vi "Test_meas_mode_status.vi"() -> ()   [LabVIEW 2019]
uses:
  D:/SOFT_REPO_GUM/renishawxl80sdk/XL-80_forum DLL/Interop.DX10SDKADAPTORLib.dll
  SOFT_REPO_GUM/renishawxl80sdk/XL-80_forum DLL/Interop.DX10SDKADAPTORLib.dll
panel:
  out "32bit integer":i32
  out "MEASUREMENT_INDETERMINATE":i32(ring) items=["MEASUREMENT_INDETERMINATE", "MEASUREMENT_LINEAR_PLANE", "MEASUREMENT_LINEAR_RETRO", "MEASUREMENT_ANGULAR", "MEASUREMENT_STRAIGHTNESS_SHORT", "MEASUREMENT_STRAIGHTNESS_LONG", "MEASUREMENT_VELOCITY_RETRO"]
  out "x << y":u32
  out "modeMask":u32
  out "status":u32
  out "ML10_MEASUREMENT_MODE":i32(ring)=1 items=["ML10_AVERAGING_ON"=1, "ML10_TPIN_SELECTED"=4, "ML10_BEAM_LOW"=64, "ML10_BEAM_LOSS"=128, "ML10_STABILITY_LOSS"=256, "ML10_PREHEAT"=2048, "ML10_LASER_TOO_COLD"=4096, "ML10_LASER_TOO_HOT"=8192, "ML10_LASER_UNSTABLE"=16384, "ML10_LASER_FAIL"=32768, "ML10_NOT_RESPONDING"=65536, "ML10_LONG_TERM_AVERAGING_ON"=524288, "ML10_MEASUREMENT_MODE"=7340032, "ML10_HIGH_SPEED_ERROR"=8388608, "ML10_DYNAMIC_SELECTED"=16777216]
  out "Status":i32(ring)=1 items=["ML10_AVERAGING_ON"=1, "ML10_TPIN_SELECTED"=4, "ML10_BEAM_LOW"=64, "ML10_BEAM_LOSS"=128, "ML10_STABILITY_LOSS"=256, "ML10_PREHEAT"=2048, "ML10_LASER_TOO_COLD"=4096, "ML10_LASER_TOO_HOT"=8192, "ML10_LASER_UNSTABLE"=16384, "ML10_LASER_FAIL"=32768, "ML10_NOT_RESPONDING"=65536, "ML10_LONG_TERM_AVERAGING_ON"=524288, "ML10_MEASUREMENT_MODE"=7340032, "ML10_HIGH_SPEED_ERROR"=8388608, "ML10_DYNAMIC_SELECTED"=16777216]
  out "pbstrSerNum":string
  out "Connect":bool
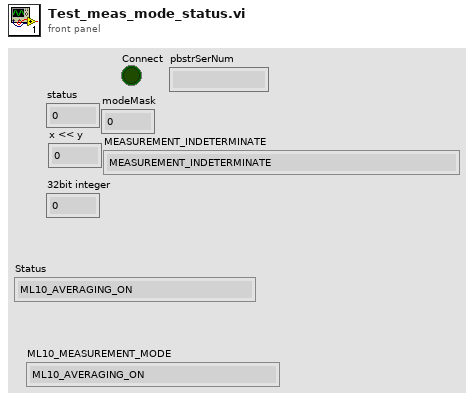
[diagram p1: front panel]
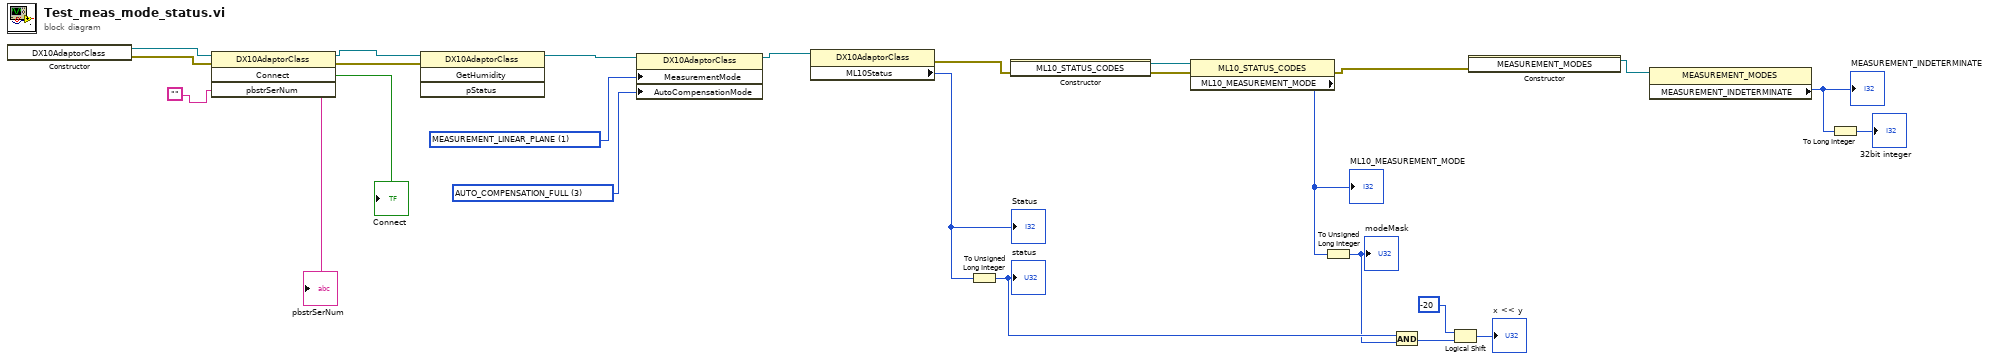
[diagram p0: block diagram]
diagram:
  w18 = 3 items=["AUTO_COMPENSATION_OFF"=0, "AUTO_COMPENSATION_AIR"=1, "AUTO_COMPENSATION_FULL"=3] ("AutoCompensationMode")
  w19 = 1 items=["MEASUREMENT_INDETERMINATE", "MEASUREMENT_LINEAR_PLANE", "MEASUREMENT_LINEAR_RETRO", "MEASUREMENT_ANGULAR", "MEASUREMENT_STRAIGHTNESS_SHORT", "MEASUREMENT_STRAIGHTNESS_LONG", "MEASUREMENT_VELOCITY_RETRO"] ("MeasurementMode")
  n1 = constructor class="DX10AdaptorClass"() -> (reference out=w16:refnum<k24>, error out=w25:errorcluster)  [unwired: 3 in, 1 out]
  n2 = invoke class="DX10AdaptorClass" method="Connect"(reference=w16, error in=w25, "pbstrSerNum"="") -> (reference out=w15:refnum<k24>, error out=w21:errorcluster, "Connect"=→"Connect":bool, "pbstrSerNum"=→"pbstrSerNum":string)  [unwired: 1 in]
  n3 = invoke class="DX10AdaptorClass" method="GetHumidity"(reference=w15, error in=w21) -> (reference out=w20:refnum<k24>)  [unwired: 2 in, 3 out]
  n4 = property class="DX10AdaptorClass"(reference=w20, "MeasurementMode"=w19, "AutoCompensationMode"=w18) -> (reference out=w17:refnum<k24>)  [unwired: 1 in, 1 out]
  n5 = property class="DX10AdaptorClass"(reference=w17) -> (error out=w14:errorcluster, "ML10Status"=w11:i32)  [unwired: 1 in, 1 out]
  "Status" <- w11
  n6 = To Unsigned Long Integer(number=w11) -> (unsigned 32bit integer=w9:u32)
  "status" <- w9
  n7 = constructor class="ML10_STATUS_CODES"(error in=w14) -> (reference out=w13:refnum<k24>, error out=w12:errorcluster)  [unwired: 2 in, 1 out]
  n8 = property class="ML10_STATUS_CODES"(reference=w13, error in=w12) -> (error out=w4:errorcluster, "ML10_MEASUREMENT_MODE"=w10:i32)  [unwired: 1 out]
  "ML10_MEASUREMENT_MODE" <- w10
  n9 = To Unsigned Long Integer(number=w10) -> (unsigned 32bit integer=w8:u32)
  "modeMask" <- w8
  n10 = And(x=w9, y=w8) -> (x .and. y?=w7:u32)
  n11 = Logical Shift(y=i16 -20, x=w7) -> (x << y=→"x << y":u32)
  n12 = constructor class="MEASUREMENT_MODES"(error in=w4) -> (reference out=w3:refnum<k24>)  [unwired: 2 in, 2 out]
  n13 = property class="MEASUREMENT_MODES"(reference=w3) -> ("MEASUREMENT_INDETERMINATE"=w2:i32)  [unwired: 1 in, 2 out]
  "MEASUREMENT_INDETERMINATE" <- w2
  n14 = To Long Integer(number=w2) -> (32bit integer=→"32bit integer":i32)
